vi "Periodic Tasks.vi"(8 "error in":errorcluster) -> ()   [LabVIEW 2020]
doc: "This VI runs in parallel to other robot code. It can contain as many user-defined periodic loops as you need. These can carry out PID or other sorts of timed response."
uses:
  <vilib>/Rock Robotics/WPI/Utilities/WPI_GetSetVariantRefNum.vi
  <vilib>/Rock Robotics/Network Tables/NT Read Boolean.vi
  Drive/Implementation/Infrastructure/Drive Command Helper.vi
  <vilib>/Rock Robotics/Network Tables/NT Write Boolean.vi
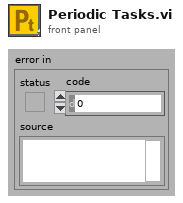
[diagram p1: front panel]
types:
  T1 = typedef "WPI_JoystickDevRef.ctl" = cluster{"Device":T2}
  T2 = typedef "WPI_JoystickDeviceEnum.ctl" = enum16{"USB 0", "USB 1", "USB 2", "USB 3", "USB 4", "USB 5"}
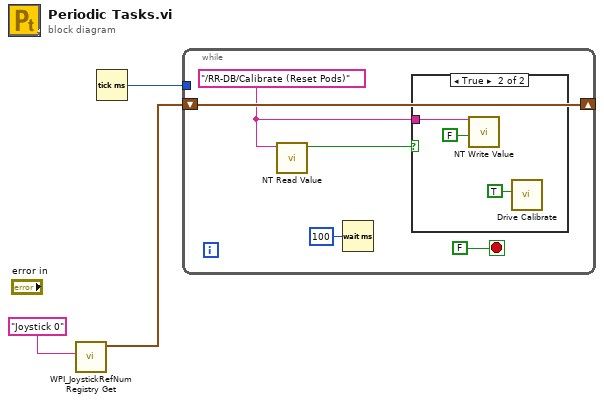
[diagram p0: block diagram]
diagram:
  n1 = call <vilib>:"WPI_JoystickRefNum Registry Get.vi"("refnum name"="Joystick 0") -> ("JoystickDevRef"=w2:T1)  [unwired: 1 in, 9 out]
  n2 = Tick Count (ms)() -> (millisecond timer value=w1:u32)
  n3 = while {
    shift-right: [w7] -> _
    shift-left: w2 -> [w7]
    tunnel: w1 -> [_]
    stop <- FALSE stop-if-true
    w4 = "/RR-DB/Calibrate (Reset Pods)" ("Name")
    n4 = call-poly <vilib>:"NT Read Value.vi"("Name"=w4) -> ("Boolean"=w5:bool)  [unwired: 9 in, 1 out]
    n5 = Wait (ms)(milliseconds to wait=u32 100) -> ()  [unwired: 1 out]
    n6 = case shown="True" w5 {
      tunnel: w4 -> [_ w10]
      frame False {
      }
      frame True {
        n7 = call-poly <vilib>:"NT Write Value.vi"("Boolean"=FALSE, "Name"=w10) -> ()  [unwired: 9 in, 1 out]
        n8 = call "Drive Calibrate.vi"("reset pods"=TRUE) -> ()  [unwired: 10 in, 1 out]
      }
    }
  }
